vi "Print.vi"(10 "String":string, 11 "OT3IPrinter In":refnum<class "OT3IPrinter.lvclass">) -> (3 "OT3IPrinter Out":refnum<class "OT3IPrinter.lvclass">)   [LabVIEW 2018, in "OfficeTron3000.lvlib" / "OT3IPrinter.lvclass"]
uses:
  OT3IPrinter.lvclass
  OT3IPrinter.lvclass/OT3IPrinter.ctl
  OfficeTron3000/OfficeTron3000.lvclass
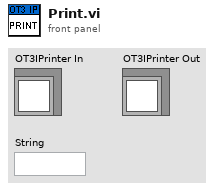
[diagram p1: front panel]
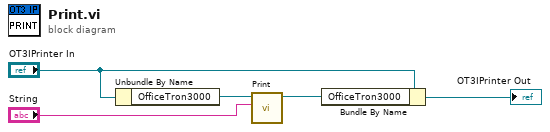
[diagram p0: block diagram]
diagram:
  n1 = Unbundle By Name("OT3IPrinter In") -> ("OfficeTron3000"=w3:refnum<class "OfficeTron3000.lvclass">)
  n2 = call "Print.vi"("String"="String", "OfficeTron3000 In"=w3) -> ("OfficeTron3000 Out"=w2:refnum<class "OfficeTron3000.lvclass">)  [unwired: 9 in]
  n3 = Bundle By Name(cluster="OT3IPrinter In", "OfficeTron3000"=w2) -> (→"OT3IPrinter Out":refnum<class "OT3IPrinter.lvclass">)
